vi "DB Tools Insert Data.vi"(4 "use file? (F)":bool, 5 "create table? (F)":bool, 6 "flatten cluster? (F)":bool, 7 "data":variant, 8 "error in (no error)":errorcluster, 9 "columns":string[](array[string]), 10 "table":string, 11 "connection reference":T1) -> (0 "error out":errorcluster, 3 "connection reference out":T1)   [LabVIEW 2012, in "NI_Database_API_64.lvlib"]
doc: "Inserts a new row into the table in the database identified by the <B>connection reference</B>."
uses:
  NI_Database_API_64.lvlib
  Connection.llb/Conn ObjectReference.ctl
  Command.llb/Cmd Execute.vi
  Recordset.llb/Rec Destroy - Command.vi
  Command.llb/Cmd Delete.vi
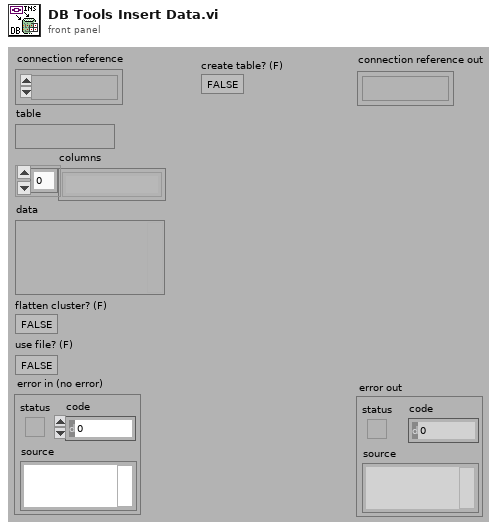
[diagram p1: front panel]
types:
  T1 = typedef "NI_Database_API_64.lvlib/Conn ObjectReference.ctl" = refnum<k1>
  T2 = typedef "NI_Database_API_64.lvlib/DB Tools Parameter Info.ctl" = cluster{"parameter name":string, "type":T3, "direction":T4, "value":variant}
  T3 = typedef "NI_Database_API_64.lvlib/DB Tools DataTypes.ctl" = enum16{"String", "Long (I32)", "Single (SGL)", "Double (DBL)", "Date/Time", "Binary"}
  T4 = typedef "NI_Database_API_64.lvlib/DB Tools Parameter Dir.ctl" = enum32{"Input", "Output", "Input/Output", "Return Value"}
  T5 = typedef "NI_Database_API_64.lvlib/Cmd ObjectReference.ctl" = refnum<k1>
  T6 = typedef "NI_Database_API_64.lvlib/Cmd-Rec Object Reference.ctl" = refnum<k1>
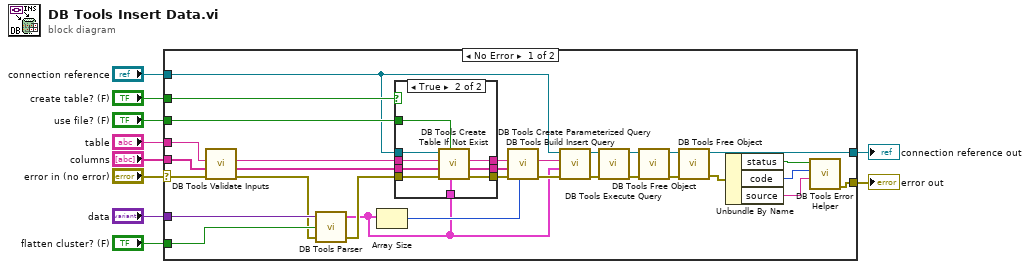
[diagram p0: block diagram]
diagram:
  n1 = case shown="No Error" "error in (no error)" {
    selector: "error in (no error)" -> [w14 w55]
    tunnel: "table" -> [w41 _]
    tunnel: [w40 w54] -> w9
    tunnel: "data" -> [w39 _]
    tunnel: "flatten cluster? (F)" -> [w38 _]
    tunnel: "create table? (F)" -> [w27 _]
    tunnel: "connection reference" -> [w13 w54]
    tunnel: "columns" -> [w21 _]
    tunnel: [w19 w55] -> w3
    tunnel: "use file? (F)" -> [w15 _]
    frame No Error {
      n2 = call "DB Tools Validate Inputs.vi"("error in (no error)"=w14, "columns"=w21, "table"=w41) -> ("error out"=w11:errorcluster, "columns out"=w12:string[], "table out"=w26:string)  [unwired: 2 in]
      n3 = call "DB Tools Parser.vi"("error in (no error)"=w11, "flatten cluster? (F)"=w38, "variant"=w39) -> ("error out"=w25:errorcluster, "parameters"=w24:T2[])  [unwired: 1 in]
      n4 = Array Size(array=w24) -> (size(s)=w29:i32)
      n5 = case shown="True" w27 {
        tunnel: [w43 w53] -> w28
        tunnel: w26 -> [w44 w52]
        tunnel: w12 -> [w42 w46]
        tunnel: w25 -> [w43 w51]
        tunnel: w24 -> [_ w47]
        tunnel: [w44 w50] -> w23
        tunnel: w13 -> [_ w49]
        tunnel: [w42 w48] -> w22
        tunnel: w15 -> [_ w45]
        frame False {
        }
        frame True {
          n6 = call "DB Tools Create Table If Not Exist.vi"("parameters"=w47, "use file? (F)"=w45, "error in (no error)"=w51, "columns"=w46, "table name"=w52, "connection reference"=w49) -> ("error out"=w53:errorcluster, "columns out"=w48:string[], "table name out"=w50:string)  [unwired: 1 out]
        }
      }
      n7 = call "DB Tools Build Insert Query.vi"("num parameters"=w29, "error in (no error)"=w28, "columns"=w22, "table name"=w23) -> ("error out"=w30:errorcluster, "insert query"=w31:string)  [unwired: 3 in]
      n8 = call "DB Tools Create Parameterized Query.vi"("error in (no error)"=w30, "parameters"=w24, "SQL query"=w31, "connection reference"=w13) -> ("error out"=w36:errorcluster, "command reference"=w35:T5)  [unwired: 3 in, 1 out]
      n9 = call-poly "DB Tools Execute Query.vi"("error in (no error)"=w36, "command reference"=w35) -> ("error out"=w33:errorcluster, "command-recordset reference"=w34:T6)  [unwired: 6 in]
      n10 = call-poly "DB Tools Free Object.vi"("error in (no error)"=w33, "command-recordset reference"=w34) -> ("error out"=w37:errorcluster, "command reference"=w32:T5)  [unwired: 8 in]
      n11 = call-poly "DB Tools Free Object.vi"("error in (no error)"=w37, "command reference"=w32) -> ("error out"=w16:errorcluster, "connection reference"=w40:T1)  [unwired: 8 in]
      n12 = Unbundle By Name(w16) -> ("status"=w20:bool, "code"=w17:i32, "source"=w18:string)
      n13 = call "DB Tools Error Helper.vi"("source"=w18, "code"=w17, "status"=w20) -> ("error out"=w19:errorcluster)  [unwired: 8 in]
    }
    frame Error {
    }
  }
  "error out" <- w3
  "connection reference out" <- w9
